vi "testSetLvLib.vi"(8 "error in (no error)":errorcluster) -> (0 "error out":errorcluster)   [LabVIEW 2018]
uses:
  src/LibReader/LibReader.lvclass
  src/LibReader/LibReader.lvclass/LibReader.ctl
  <vilib>/addons/_JKI Toolkits/Caraya/classes/Assert/Assert Equal Value_Variant.vi
  <vilib>/addons/_JKI Toolkits/Caraya/classes/Assert/Assert True.vi
  <vilib>/addons/_JKI Toolkits/Caraya/classes/Assert/Assert Error.vi
  <vilib>/addons/_JKI Toolkits/Caraya/classes/Test/Test.lvclass
  <vilib>/addons/_JKI Toolkits/Caraya/classes/Assert/Assert.lvclass
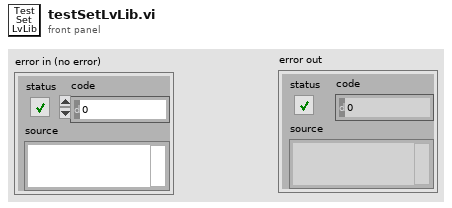
[diagram p1: front panel]
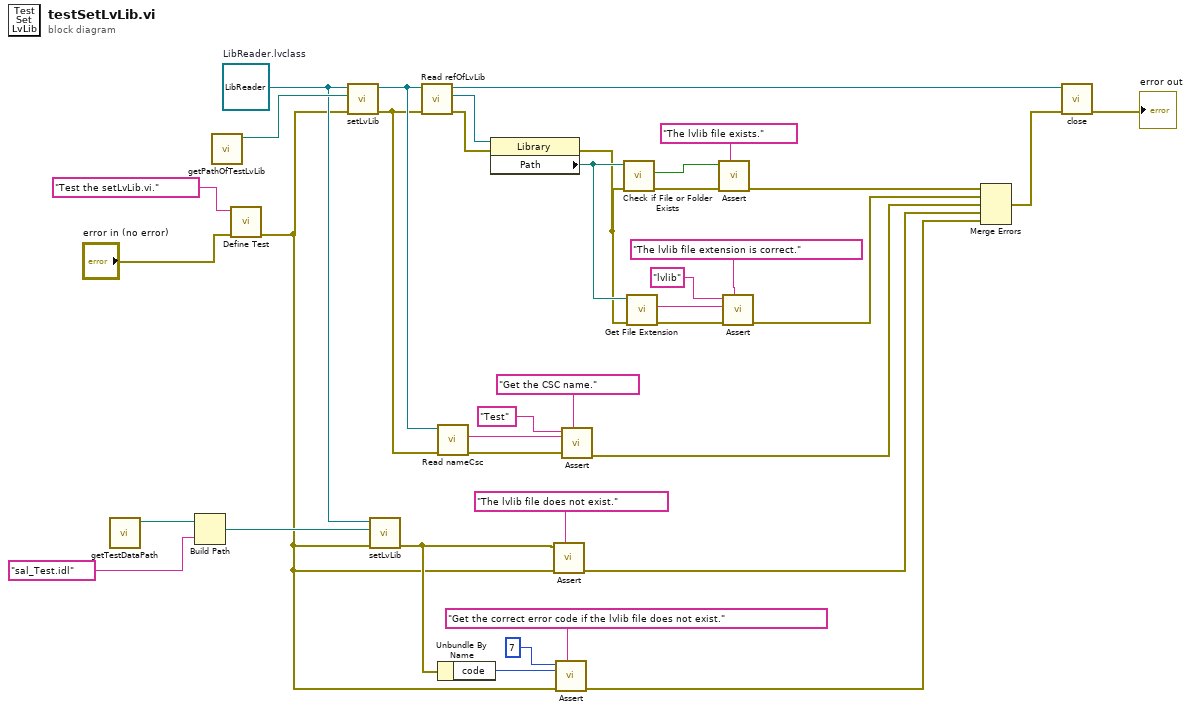
[diagram p0: block diagram]
diagram:
  w20 = refnum<class "LibReader.lvclass"> refnum  # LibReader.lvclass
  n1 = call "getTestDataPath.vi"() -> ("testDataPath"=w19:path)  [unwired: 11 in]
  n2 = Build Path(base path=w19, name or relative path="sal_Test.idl") -> (appended path=w17:path)
  n3 = call "getPathOfTestLvLib.vi"() -> ("testLvLibPath"=w38:path)  [unwired: 11 in]
  n4 = call <vilib>:"Define Test.vi"("error in (no error)"="error in (no error)", "Label (VI Title)"="Test the setLvLib.vi.") -> ("error out"=w13:errorcluster)  [unwired: 9 in]
  n5 = call "setLvLib.vi"("error in (no error)"=w13, "pathLvLib"=w38, "LibReader in"=w20) -> ("error out"=w9:errorcluster, "LibReader out"=w10:refnum<class "LibReader.lvclass">)  [unwired: 7 in]
  n6 = call "setLvLib.vi"("error in (no error)"=w13, "pathLvLib"=w17, "LibReader in"=w20) -> ("error out"=w15:errorcluster)  [unwired: 7 in, 1 out]
  n7 = call "Read refOfLvLib.vi"("error in (no error)"=w9, "LibReader in"=w10) -> ("error out"=w33:errorcluster, "refOfLvLib"=w36:refnum<vi>, "LibReader out"=w37:refnum<class "LibReader.lvclass">)  [unwired: 7 in]
  n8 = call "Read nameCsc.vi"("error in (no error)"=w9, "LibReader in"=w10) -> ("error out"=w8:errorcluster, "nameCsc"=w7:string)  [unwired: 7 in, 1 out]
  n9 = Unbundle By Name(w15) -> ("code"=w14:i32)
  n10 = property class="Library"(reference=w36, error in=w33) -> (error out=w31:errorcluster, "Path"=w32:path)  [unwired: 1 out]
  n11 = call-poly <vilib>:"Assert.vi"("Label"="The lvlib file does not exist.", "error in (no error)"=w13, "Error?"=w15) -> ("error out"=w2:errorcluster)  [unwired: 8 in]
  n12 = call-poly <vilib>:"Assert.vi"("Label"="Get the correct error code if the lvlib file does not exist.", "error in (no error)"=w13, "Y"=w14, "X"=7) -> ("error out"=w3:errorcluster)  [unwired: 7 in]
  n13 = call-poly <vilib>:"Assert.vi"("Label"="Get the CSC name.", "error in (no error)"=w8, "Y"=w7, "X"="Test") -> ("error out"=w1:errorcluster)  [unwired: 7 in]
  n14 = call <vilib>:"Check if File or Folder Exists.vi"("error in (no error)"=w31, "path"=w32) -> ("error out"=w30:errorcluster, "file or folder exists?"=w29:bool)  [unwired: 7 in, 1 out]
  n15 = call <vilib>:"Get File Extension.vi"("error in (no error)"=w31, "file"=w32) -> ("error out"=w27:errorcluster, "lowercase file extension"=w26:string)  [unwired: 5 in, 3 out]
  n16 = call-poly <vilib>:"Assert.vi"("Label"="The lvlib file exists.", "error in (no error)"=w30, "True?"=w29) -> ("error out"=w24:errorcluster)  [unwired: 8 in]
  n17 = call-poly <vilib>:"Assert.vi"("Label"="The lvlib file extension is correct.", "error in (no error)"=w27, "Y"=w26, "X"="lvlib") -> ("error out"=w23:errorcluster)  [unwired: 7 in]
  n18 = Merge Errors(w24, w23, w1, w2, w3) -> (w22:errorcluster)
  n19 = call "close.vi"("error in (no error)"=w22, "LibReader in"=w37) -> ("error out"=→"error out":errorcluster)  [unwired: 8 in, 1 out]
